vi "Keithley 2002 Calc Read.vi"(2 "error in":T1, 3 "read source (calc1:0)":u16(ring) items=["calc 1", "calc 2", "calc 3"], 4 "GPIB address":string="16") -> (0 "error out":T1, 1 "result":dbl format="%.6e")   [LabVIEW 2020]
doc: "This VI is used to read the results of the selected calculation. The calculations are configured using the Calc1,2, or 3 Config VI's.\n\nThese calculations do not show up in the other read VI's."
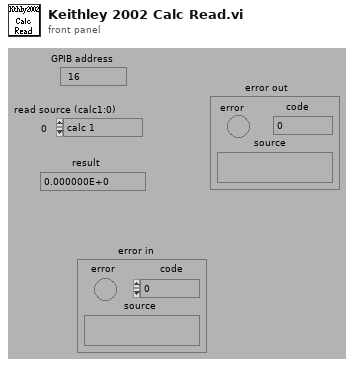
[diagram p1: front panel]
types:
  T1 = cluster{"error":bool, "code":i32, "source":string}
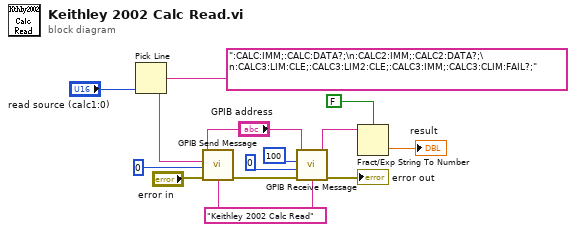
[diagram p0: block diagram]
diagram:
  w4 = "Keithley 2002 Calc Read"
  n1 = Pick Line(multi-line string=":CALC:IMM;:CALC:DATA?;\n:CALC2:IMM;:CALC2:DATA?;\n:CALC3:LIM:CLE;:CALC3:LIM2:CLE;:CALC3:IMM;:CALC3:CLIM:FAIL?;", line index="read source (calc1:0)") -> (output string=w10:string)  [unwired: 1 in]
  n2 = call "GPIB Send Message.vi"("address string"="GPIB address", "write buffer"=w10, "source"=w4, "write mode (set END:0)"=0, "error in"="error in") -> ("error out"=w8:T1)  [unwired: 2 in, 2 out]
  n3 = call "GPIB Receive Message.vi"("address string"="GPIB address", "byte count"=100, "source"=w4, "read mode"=0, "error in"=w8) -> ("read buffer"=w3:string, "error out"=→"error out":T1)  [unwired: 2 in, 1 out]
  n4 = Fract/Exp String To Number(use system decimal point (T)=FALSE, string=w3) -> (number=→"result":dbl)  [unwired: 2 in, 1 out]
